vi "Set_Time_2.vi"() -> ()   [LabVIEW 2021]
uses:
  <vilib>/nisyscfg/Close (System).vi
  <vilib>/nisyscfg/nisyscfg.lvlib
panel:
  in  "restart RT?":bool
  out "PC current time":timestamp
  in  "Session in (localhost)":refnum<k21>="localhost"
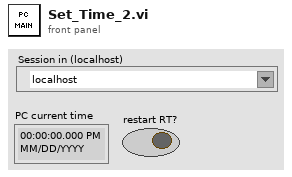
[diagram p1: front panel]
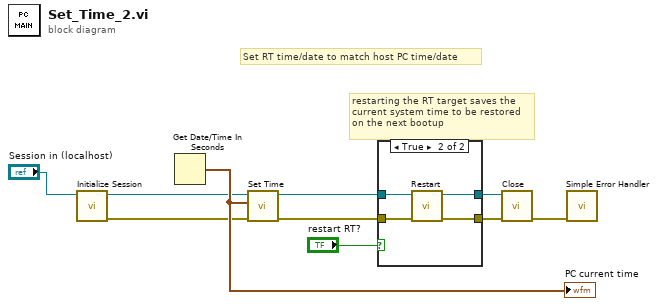
[diagram p0: block diagram]
diagram:
  # "restarting the RT target saves the\ncurrent system time to be restored\non the next bootup"
  # "Set RT time/date to match host PC time/date"
  n1 = call <vilib>:"Initialize Session.vi"("Target (localhost)"="Session in (localhost)") -> ("error out"=w2:errorcluster, "Session out"=w1:refnum<k21>)  [unwired: 9 in]
  n2 = Get Date/Time In Seconds() -> (seconds since 1Jan1904=w10:timestamp)
  "PC current time" <- w10
  n3 = call <vilib>:"Set Time.vi"("error in (no error)"=w2, "Time"=w10, "Session in (localhost)"=w1) -> ("error out"=w9:errorcluster, "Session out"=w8:refnum<k21>)  [unwired: 5 in, 2 out]
  n4 = case shown="True" "restart RT?" {
    tunnel: w9 -> [w12 w16]
    tunnel: w8 -> [w11 w15]
    tunnel: [w12 w14] -> w7
    tunnel: [w11 w13] -> w5
    frame False {
    }
    frame True {
      n5 = call <vilib>:"Restart.vi"("error in (no error)"=w16, "Session in"=w15) -> ("error out"=w14:errorcluster, "Session out"=w13:refnum<k21>)  [unwired: 7 in, 1 out]
    }
  }
  n6 = call-poly <vilib>:"Close.vi"("error in (no error)"=w7, "Session in"=w5) -> ("error out"=w6:errorcluster)  [unwired: 9 in]
  n7 = call <vilib>:"Simple Error Handler.vi"("error in (no error)"=w6) -> ()  [unwired: 4 in, 5 out]
